vi "Init Hardware.vi"(8 "error in (no error)":errorcluster, 11 "Keithley in":refnum<class "Keithley Driver.lvclass">) -> (0 "error out":errorcluster, 3 "Keithley out":refnum<class "Keithley Driver.lvclass">)   [LabVIEW 2016, in "Keithley Driver.lvclass"]
uses:
  Keithley Driver.lvclass
  C:/github/NHMFL_Core/Libraries/Instruments/Instrument Driver/Instrument Driver.lvclass
  C:/github/NHMFL_Core/Libraries/Instruments/VISA Instrument/VISA Instrument.lvclass
  Instrument Driver/Instrument Driver.lvclass/Instrument Driver.ctl
  VISA Instrument/VISA Instrument.lvclass/VISA Instrument.ctl
  Instrument Driver/Read Recorder name.vi
  VISA Instrument/Read VISA resource.vi
  Instrument Driver/Write Channel names.vi
  Instrument Driver/Write Channel units.vi
  VISA Instrument/Write VISA resource.vi
  Read Keithley user configuration.vi
  GPIB/VISA  Send Receive.vi
  Simple VISA Reader/Simple VISA Reader Driver.lvclass
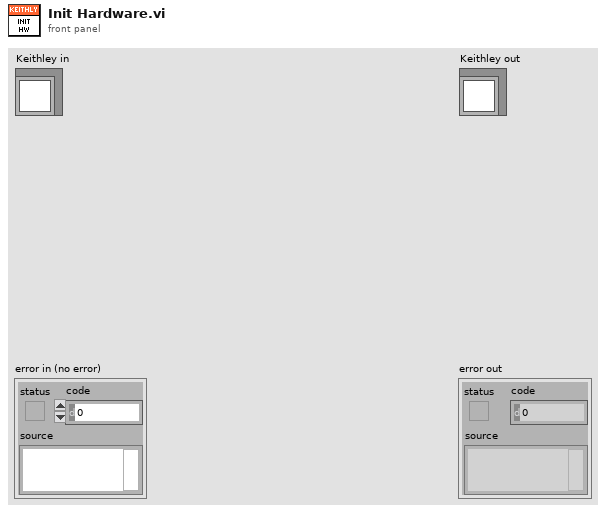
[diagram p1: front panel]
types:
  T1 = typedef "Keithley Meter Parameters.ctl" = cluster{"Range (-1: auto)":dbl, "Integration Time (NPLCs)":dbl, "Function":T2, "W Offset comp":bool, "4-wire W":bool, "Scale":dbl, "Offset":dbl}
  T2 = typedef "KeithleyMeter Function.ctl" = enum16{"VOLTAGE", "CURRENT", "RESISTANCE"}
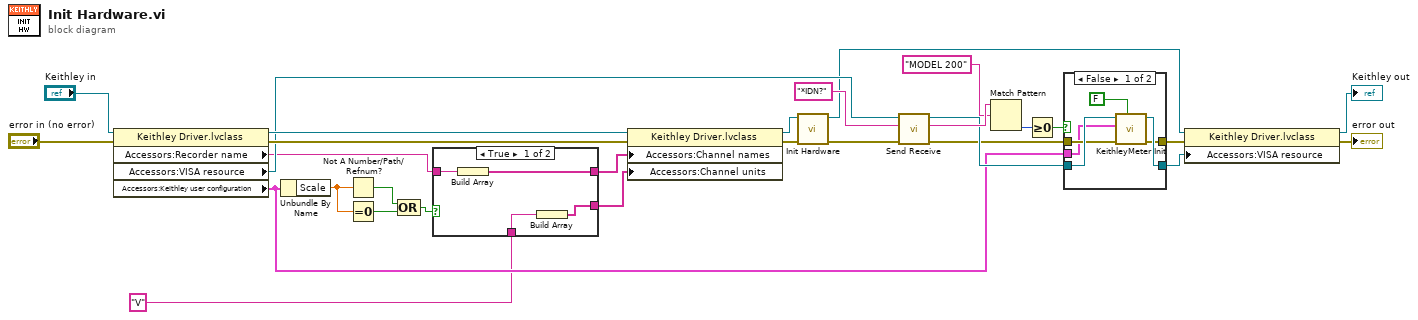
[diagram p0: block diagram]
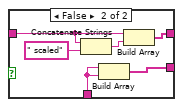
[diagram p2: hidden frame]
diagram:
  n1 = property class="Keithley Driver.lvclass"(reference="Keithley in", error in="error in (no error)") -> (reference out=w29:refnum<class "Keithley Driver.lvclass">, error out=w28:errorcluster, "Accessors:Recorder name"=w4:string, "Accessors:VISA resource"=w23:refnum<visa-resource-name>, "Accessors:Keithley user configuration"=w5:T1)
  n2 = Unbundle By Name(w5) -> ("Scale"=w6:dbl)
  n3 = Not A Number/Path/Refnum?(number/path/refnum=w6) -> (NaN/Path/Refnum?=w9:bool)
  n4 = Equal To 0?(x=w6) -> (x = 0?=w8:bool)
  n5 = Compound Arithmetic op=OR(w9, w8) -> (w7:bool)
  n6 = case shown="True" w7 {
    tunnel: w4 -> [w33 w38]
    tunnel: [w32 w39] -> w3
    tunnel: [w30 w35] -> w2
    tunnel: "V" -> [w31 w34]
    frame True {
      n7 = Build Array(w33) -> (w32:string[])
      n8 = Build Array(w31) -> (w30:string[])
    }
    frame False {
      n9 = Concatenate Strings(w38, " scaled" ("string")) -> (w36:string)
      n10 = Build Array(w34, w34) -> (w35:string[])
      n11 = Build Array(w38, w36) -> (w39:string[])
    }
  }
  n12 = property class="Keithley Driver.lvclass"(reference=w29, error in=w28, "Accessors:Channel names"=w3, "Accessors:Channel units"=w2) -> (reference out=w24:refnum<class "Keithley Driver.lvclass">, error out=w26:errorcluster)
  n13 = call-parent "Init Hardware.vi"("error in (no error)"=w26, "Instrument Driver in"=w24) -> ("error out"=w16:errorcluster, "Instrument Driver out"=w12:refnum<class "Keithley Driver.lvclass">)  [unwired: 8 in]
  n14 = call-poly "Send Receive.vi"("error in (no error)"=w16, "data string in"="*IDN?", "VISA Resource Name"=w23) -> ("error out"=w15:errorcluster, "data string out"=w21:string, "VISA Resource Name Out"=w17:refnum<visa-resource-name>)  [unwired: 6 in]
  n15 = Match Pattern(string=w21, regular expression="MODEL 200") -> (offset past match=w19:i32)  [unwired: 1 in, 3 out]
  n16 = Greater Or Equal To 0?(x=w19) -> (x >= 0?=w18:bool)
  n17 = case shown="False" w18 {
    tunnel: w17 -> [w45 w47]
    tunnel: w15 -> [w44 w46]
    tunnel: [w43 w47] -> w14
    tunnel: [w42 w46] -> w13
    tunnel: w5 -> [w41 _]
    frame False {
      n18 = call "KeithleyMeter Init.vi"("Source-meter"=FALSE, "Error In"=w44, "Parameters"=w41, "VISA resource name"=w45) -> ("Error Out"=w42:errorcluster, "VISA resource name out"=w43:refnum<visa-resource-name>)  [unwired: 6 in]
    }
    frame True {
    }
  }
  n19 = property class="Keithley Driver.lvclass"(reference=w12, error in=w13, "Accessors:VISA resource"=w14) -> (reference out=→"Keithley out":refnum<class "Keithley Driver.lvclass">, error out=→"error out":errorcluster)
